vi "Set Slave Address.vi"(8 "error in":errorcluster, 11 "Red-y Read Write CFG in":refnum<class "Red-y Pressure Control CFG.lvclass">) -> (0 "error out":errorcluster, 3 "Red-y Read Write CFG out":refnum<class "Red-y Pressure Control CFG.lvclass">)   [LabVIEW 2023, in "Red-y Pressure Control CFG.lvclass"]
uses:
  Red-y Pressure Control CFG.lvclass
  Configuration/Configuration JSON/Configuration JSON Base/CFG JSON.lvclass/CFG JSON.ctl
  Red-y Pressure Control CFG.lvclass/Red-y Pressure Control CFG.ctl
  909555fc-04ff-413f-956c-db7b5203db77.vi
  <vilib>/JDP Science/JSONtext/Find Item.vi
  <vilib>/JDP Science/JSONtext/Next JSON Value.vi
  <vilib>/JDP Science/JSONtext/String Subset.vi
  <vilib>/JDP Science/JSONtext/Parsing/Advance past next JSON Value (inlined COPY).vi
  <vilib>/JDP Science/JSONtext/Parsing/Advance past whitespace.vi
  <vilib>/JDP Science/JSONtext/Parsing/Advance past String.vi
  <vilib>/JDP Science/JSONtext/Parsing/Advance past Number.vi
  <vilib>/JDP Science/JSONtext/Parsing/Advance past Line Ending.vi
  <vilib>/JDP Science/JSONtext/Parsing/Parse Full Path or Item Name.vi
  <vilib>/JDP Science/JSONtext/Parsing/Advance past Array.vi
  <vilib>/JDP Science/JSONtext/Parsing/Advance past Object.vi
  <vilib>/JDP Science/JSONtext/support/Error Cluster From Code.vi
  <vilib>/JDP Science/JSONtext/Offset/Find Item Locations by Path.vi
  <vilib>/JDP Science/JSONtext/JSON text to Variant.vi
  <vilib>/Utility/error.llb/Error Cluster From Error Code.vi
  Voegtlin_NI_SMART_Modbus_Drivers/Low Level Driver/Modbus Write U16.vi
  <vilib>/JDP Science/JSONtext/LVClass Serializer/JSONtext LVClass Serializer.lvclass
  <vilib>/ErrorRing/Error Ring.xnode
  Voegtlin_NI_SMART_Modbus_Drivers/Voegtlin_NI_SMART_Modbus_Drivers.lvlib
  Configuration/Configuration JSON/Configuration JSON Base/CFG JSON.lvclass
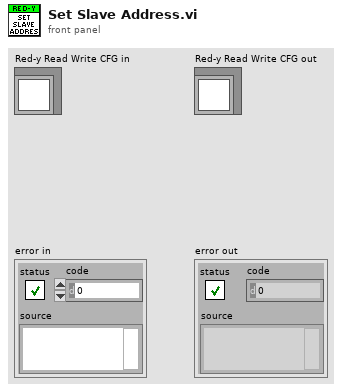
[diagram p1: front panel]
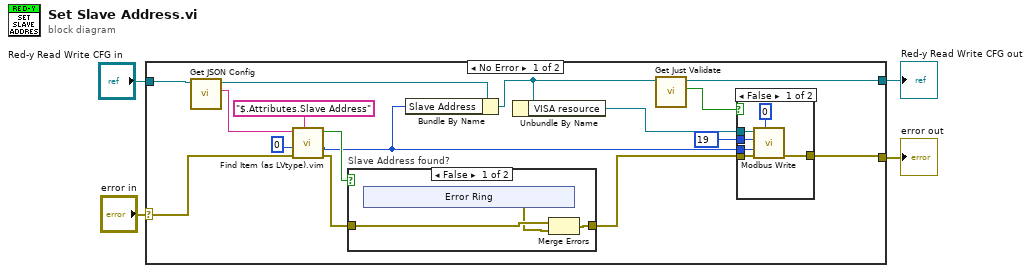
[diagram p0: block diagram]
diagram:
  n1 = case shown="No Error" "error in" {
    selector: "error in" -> [w18 w37]
    tunnel: "Red-y Read Write CFG in" -> [w20 w38]
    tunnel: [w14 w38] -> w3
    tunnel: [w17 w37] -> w2
    frame No Error {
      n2 = call "Get JSON Config.vi"("CFG Base in"=w20) -> ("<JSON>Config>"=w11:string, "CFG Base out"=w12:refnum<class "Red-y Pressure Control CFG.lvclass">)  [unwired: 9 in]
      n3 = call "Find Item (as LVtype).vim"("$Path or Item Name"="$.Attributes.Slave Address", "error in (no error)"=w18, "Data Type and Default Value"=u8 0, "JSON"=w11) -> ("error out"=w7:errorcluster, "Data"=w5:u8, "Found"=w8:bool)  [unwired: 4 in, 1 out]
      n4 = case "Slave Address found?" shown="False" w8 {
        tunnel: w7 -> [w22 w29]
        tunnel: [w23 w29] -> w6
        frame False {
          n5 = xnode "Error Ring"() -> ("error out"=w21:errorcluster)
          n6 = Merge Errors(w22, w21) -> (w23:errorcluster)
        }
        frame True {
        }
      }
      n7 = Bundle By Name(cluster=w12, "Slave Address"=w5) -> (w16:refnum<class "Red-y Pressure Control CFG.lvclass">)
      n8 = Unbundle By Name(w16) -> ("VISA resource"=w15:refnum<visa-resource-name>)
      n9 = call "Get Just Validate.vi"("CFG JSON Base in"=w16) -> ("Just Validate"=w13:bool, "CFG JSON Base out"=w14:refnum<class "Red-y Pressure Control CFG.lvclass">)  [unwired: 9 in]
      n10 = case shown="False" w13 {
        tunnel: w6 -> [w35 w36]
        tunnel: u16 19 -> [w34 _]
        tunnel: [w33 w36] -> w17
        tunnel: w5 -> [w32 _]
        tunnel: w15 -> [w31 _]
        frame False {
          n11 = call-poly "Modbus Write.vi"("Slave Address"=u8 0, "error in (no error)"=w35, "Input data U16"=w32, "Register Start Address"=w34, "VISA resource in"=w31) -> ("error out"=w33:errorcluster)  [unwired: 5 in, 1 out]
        }
        frame True {
        }
      }
    }
    frame Error {
    }
  }
  "error out" <- w2
  "Red-y Read Write CFG out" <- w3
